vi "Read FTP.vi"(8 "error in (no error)":errorcluster, 11 "FTPProtocol in":refnum<class "FTPProtocol.lvclass">) -> (0 "error out":errorcluster, 2 "FTP:FTP":refnum<class "FTP.lvclass">, 3 "FTPProtocol out":refnum<class "FTPProtocol.lvclass">)   [LabVIEW 2020, in "CSM-FileSync.lvlib" / "FTPProtocol.lvclass"]
uses:
  FTPProtocol.lvclass
  FTP Toolkit/FTP Class/FTP.lvclass
  FTPProtocol.lvclass/FTPProtocol.ctl
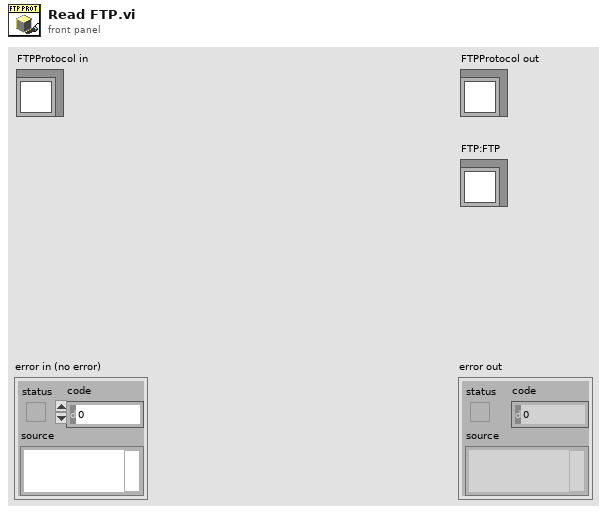
[diagram p1: front panel]
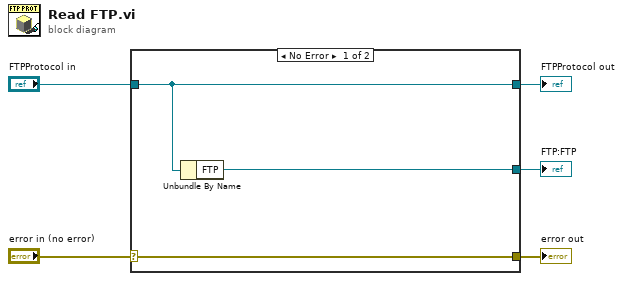
[diagram p0: block diagram]
diagram:
  n1 = case shown="No Error" "error in (no error)" {
    selector: "error in (no error)" -> [w8 w9]
    tunnel: [w8 w9] -> w4
    tunnel: [w7 w10] -> w2
    tunnel: "FTPProtocol in" -> [w7 w10]
    tunnel: [w6 _] -> w1
    frame No Error {
      n2 = Unbundle By Name(w7) -> ("FTP"=w6:refnum<class "FTP.lvclass">)
    }
    frame Error {
    }
  }
  "error out" <- w4
  "FTPProtocol out" <- w2
  "FTP:FTP" <- w1
